vi "Role Indicator.vi"(10 "Decoded Data":string[][](array[string]), 11 "NewVal":string) -> (3 "String":string)   [LabVIEW 2022 SP3]
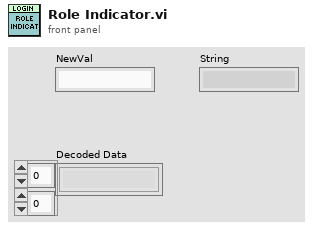
[diagram p1: front panel]
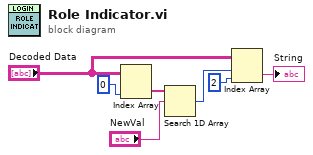
[diagram p0: block diagram]
diagram:
  n1 = Index Array(array="Decoded Data", index (col)=0 ("disabled index (col)")) -> (element=w2:string[])  [unwired: 1 in]
  n2 = Search 1D Array(1D array=w2, element="NewVal") -> (index of element=w6:i32)  [unwired: 1 in]
  n3 = Index Array(array="Decoded Data", index (row)=w6, index (col)=2) -> (element=→"String":string)
